vi "Update PAS Data By Gas.vi"(6 "pasValuesByFilter":refnum<k24>[](array[refnum]), 7 "gasID":i32, 8 "error in (no error)":errorcluster, 9 "PasDataByGas":refnum<k24>[](array[refnum]), 10 "pasDataByGas":refnum<k24>, 11 "PASData In":refnum<k24>) -> (0 "error out":errorcluster, 3 "PAS Data Out":refnum<k24>)   [LabVIEW 2015]
uses:
  C:/Distributed/CalFlex.dll
  CalFlex.dll
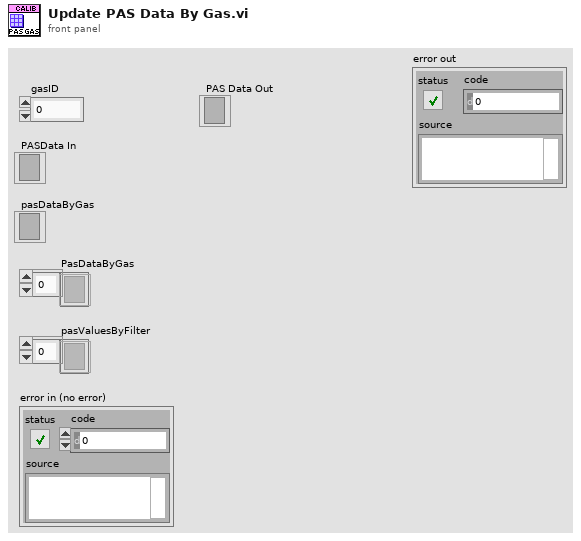
[diagram p1: front panel]
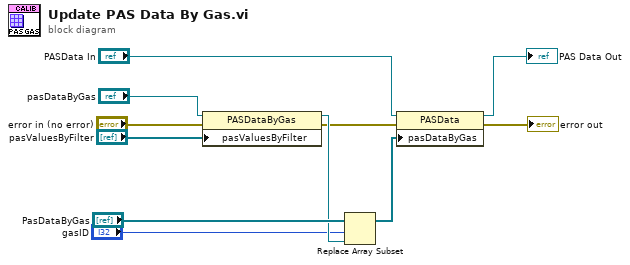
[diagram p0: block diagram]
diagram:
  n1 = property class="PASDataByGas"(reference="pasDataByGas", error in="error in (no error)", "pasValuesByFilter"="pasValuesByFilter") -> (reference out=w5:refnum<k24>, error out=w3:errorcluster)
  n2 = Replace Array Subset(array="PasDataByGas", new element=w5, index="gasID") -> (w4:refnum<k24>[])
  n3 = property class="PASData"(reference="PASData In", error in=w3, "pasDataByGas"=w4) -> (reference out=→"PAS Data Out":refnum<k24>, error out=→"error out":errorcluster)
